vi "frequency lin scan.vi"(9 "Hz/s":fxp<+/-,64,32>, 10 "Freq inc/dec":u8[](array[numeric]), 11 "Wave Reader":fxp<+/-,64,32>[](array[numeric])) -> (3 "Array":fxp<+/-,64,32>[](array[numeric]))   [LabVIEW 2020]
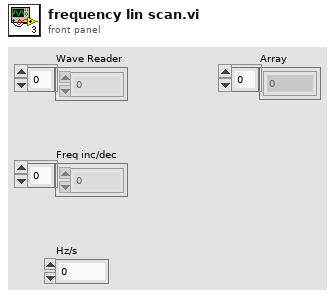
[diagram p1: front panel]
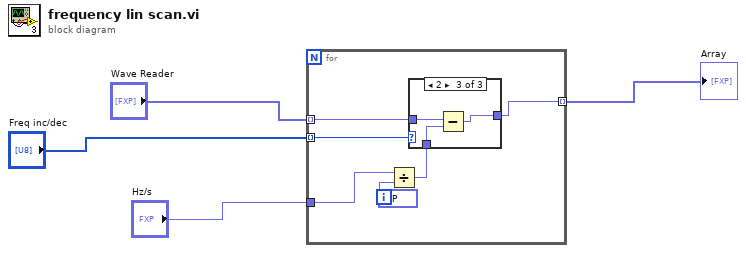
[diagram p0: block diagram]
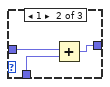
[diagram p3: hidden frame]
diagram:
  n1 = for {
    tunnel: "Hz/s" -> [w10]
    tunnel: "Wave Reader" -> [w7] mode=indexing
    tunnel: [w5] -> w3 mode=indexing
    tunnel: "Freq inc/dec" -> [w6] mode=indexing
    n2 = Divide(x=w10, y=fxp<+,20,5> 30.303009033203125) -> (x/y=w9:fxp<+/-,64,32>)
    n3 = case shown="2" w6 {
      tunnel: w7 -> [w11 w14 w17]
      tunnel: [w11 w13 w15] -> w5
      tunnel: w9 -> [_ w12 w16]
      frame 0, Default {
      }
      frame 1 {
        n4 = Add(x=w14, y=w12) -> (x+y=w13:fxp<+/-,64,32>)
      }
      frame 2 {
        n5 = Subtract(x=w17, y=w16) -> (x-y=w15:fxp<+/-,64,32>)
      }
    }
  }
  "Array" <- w3
